vi "Read Software Version.vi"(7 "Unit ID (A)":string="A", 8 "error in":errorcluster, 11 "VISA Session In":refnum<visa-resource-name>="Alicat") -> (0 "error out":errorcluster, 2 "Software Version":u8, 3 "VISA Session Out":refnum<visa-resource-name>)   [LabVIEW 2020]
doc: "Returns the software version as an integer. If the query is not valid, the VI will return a 1."
uses:
  <vilib>/Instr/_visa.llb/VISA Flush IO Buffer Mask.ctl
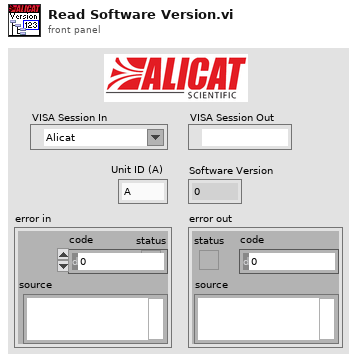
[diagram p1: front panel]
types:
  T1 = typedef "VISA Flush IO Buffer Mask.ctl" = u16
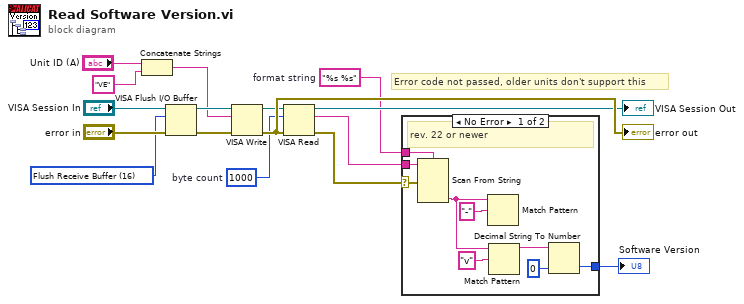
[diagram p0: block diagram]
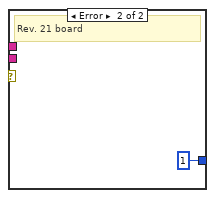
[diagram p2: hidden frame]
diagram:
  w12 = T1 16 items=["Flush Receive Buffer"=16, "Write Transmit Buffer to Device"=32, "Flush Receive Buffer (No I/O)"=64, "Flush Transmit Buffer"=128] ("Mask")
  w2 = "%s %s"  # format string
  w9 = u32 1000  # byte count
  # "Error code not passed, older units don't support this"
  n1 = Concatenate Strings("Unit ID (A)", "VE" ("string")) -> (w5:string)
  n2 = VISA Flush I/O Buffer(VISA resource name="VISA Session In", mask (16)=w12, error in (no error)="error in") -> (VISA resource name out=w14:refnum<visa-resource-name>, error out=w8:errorcluster)
  n3 = VISA Write(VISA resource name=w14, write buffer=w5, error in (no error)=w8) -> (VISA resource name out=w11:refnum<visa-resource-name>, error out=w16:errorcluster)  [unwired: 1 out]
  "error out" <- w16
  n4 = VISA Read(VISA resource name=w11, byte count=w9, error in (no error)=w16) -> (VISA resource name out=→"VISA Session Out":refnum<visa-resource-name>, read buffer=w3:string, error out=w1:errorcluster)  [unwired: 1 out]
  n5 = case shown="No Error" w1 {
    selector: w1 -> [w17 _]
    tunnel: [w21 u8 1] -> w4
    tunnel: w3 -> [w19 _]
    tunnel: w2 -> [w18 _]
    frame No Error {
      # "rev. 22 or newer"
      n6 = Scan From String(format string=w18, input string=w19, error in=w17) -> (output 2=w20:string)  [unwired: 4 in, 3 out]
      n7 = Match Pattern(string=w20, regular expression="-") -> ()  [unwired: 1 in, 4 out]
      n8 = Match Pattern(string=w20, regular expression="v") -> (before substring=w22:string)  [unwired: 1 in, 3 out]
      n9 = Decimal String To Number(string=w22, default (0L)=u8 0 ("default (0 I32)")) -> (number=w21:u8)  [unwired: 1 in, 1 out]
    }
    frame Error {
      # "Rev. 21 board"
    }
  }
  "Software Version" <- w4
